vi "DAQ Message Loop.vi"(8 "error in (no error)":errorcluster, 11 "Message Queues":T1) -> (0 "error out":errorcluster)   [LabVIEW 2018]
doc: "Message loop for handling messages pertaining to the acquisition of data from the hardware."
uses:
  <vilib>/Utility/error.llb/Error Cluster From Error Code.vi
  Hardware Configuration.ctl
  DAQ/DAQ Write.lvlib
  support/Message Queue/Message Queue.lvlib
  support/Message Queue/Enqueue Message (Single).vi
  <vilib>/ErrorRing/Error Ring.xnode
  Write State.ctl
  Write Settings Dialog.vi
  Acquisition/Task Cluster.ctl
  support/Message Queue/Message Cluster.ctl
  controls/Queue and Message Cluster.ctl
  DAQ.lvlib
  Main/Main Queue Cluster.ctl
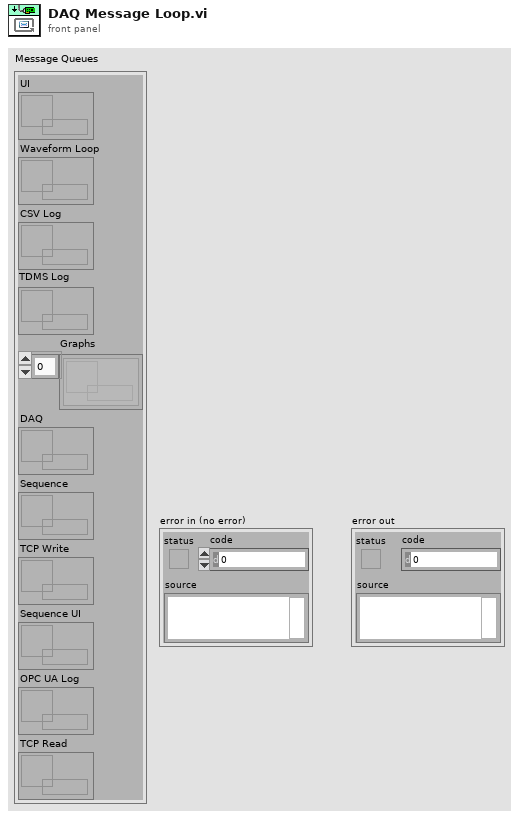
[diagram p1: front panel]
types:
  T1 = typedef "Main Queue Cluster.ctl" = cluster{"UI":refnum<queue>, "Waveform Loop":refnum<queue>, "CSV Log":refnum<queue>, "TDMS Log":refnum<queue>, "Graphs":refnum<queue>[], "DAQ":refnum<queue>, "Sequence":refnum<queue>, "TCP Write":refnum<queue>, "Sequence UI":refnum<queue>, "OPC UA Log":refnum<queue>, "TCP Read":refnum<queue>}
  T2 = typedef "DAQ.lvlib/DAQ Write.lvlib/Hardware Configuration.ctl" = cluster{"Tasks":T3[]}
  T3 = typedef "Task Cluster.ctl" = cluster{"DAQmx Task":refnum<k21>, "Read-Write Radio":enum32{"Read", "Write"}}
  T4 = typedef "Queue and Message Cluster.ctl" = cluster{"return Message Queue":refnum<queue>, "Message":string, "Variant":variant}
  T5 = typedef "Write State.ctl" = enum16{"Idle", "Writting"}
  T6 = typedef "Message Queue.lvlib/Message Cluster.ctl" = cluster{"Message":string, "Message Data":variant}
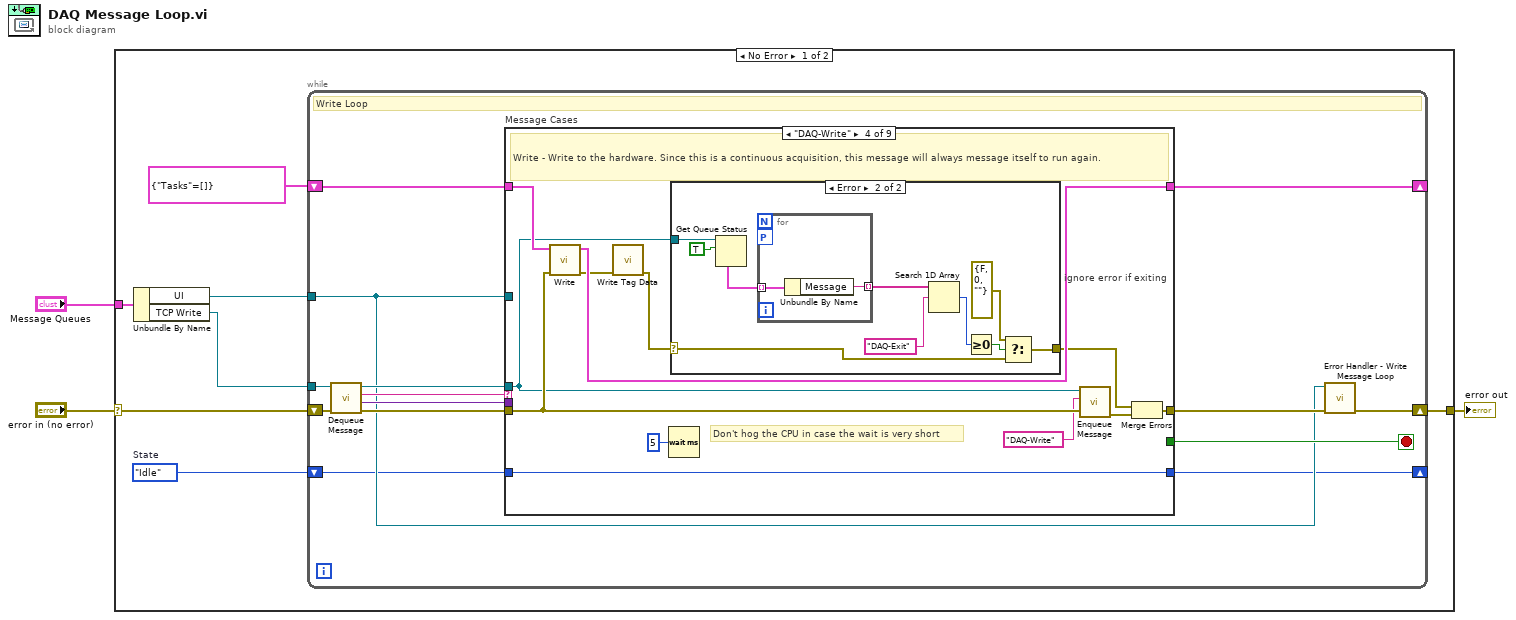
[diagram p0: block diagram]
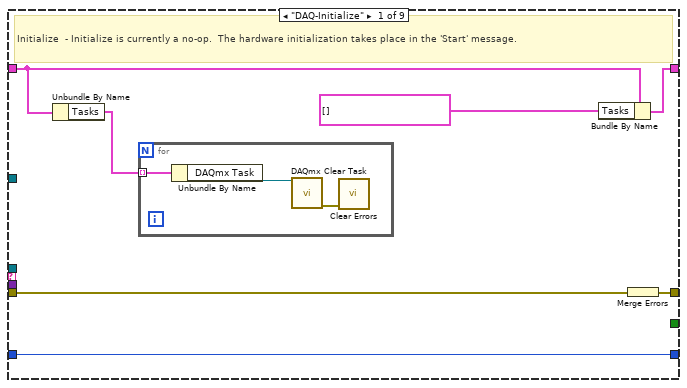
[diagram p2: hidden frame]
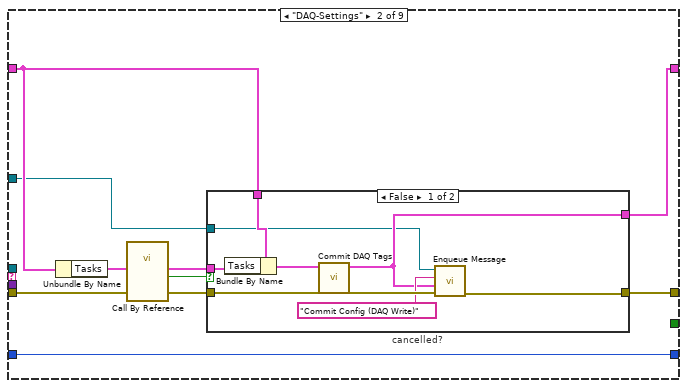
[diagram p3: hidden frame]
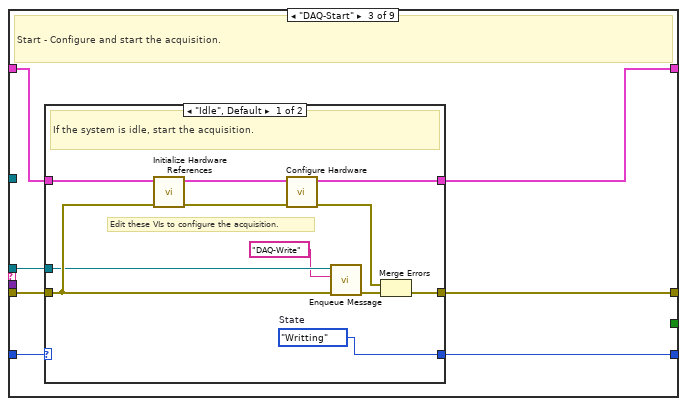
[diagram p5: hidden frame]
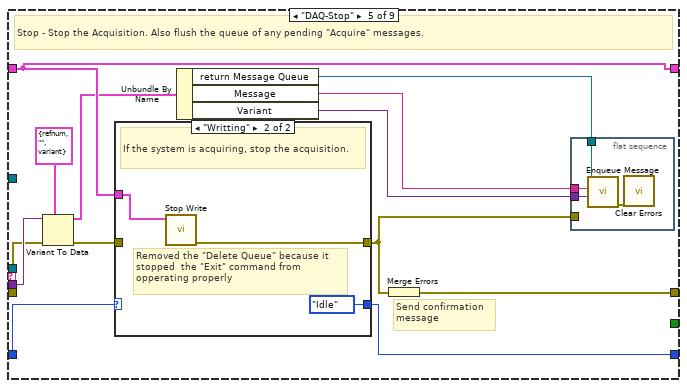
[diagram p8: hidden frame]
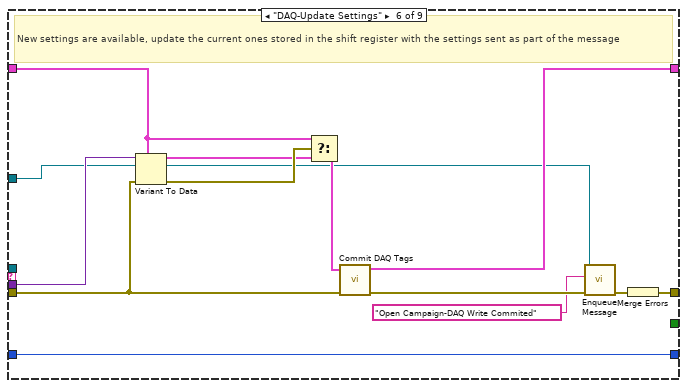
[diagram p10: hidden frame]
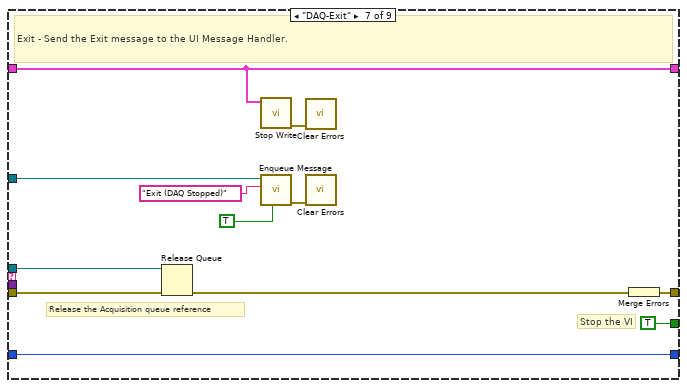
[diagram p11: hidden frame]
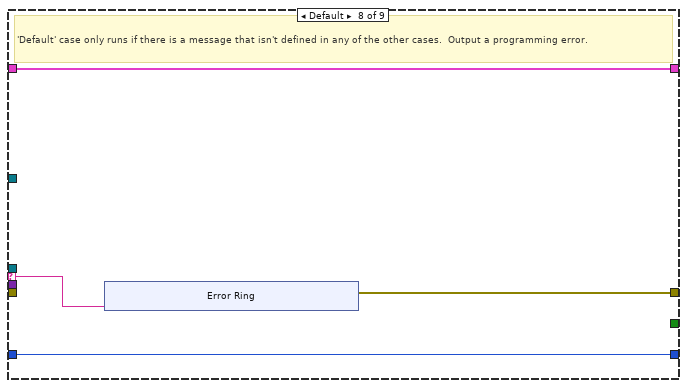
[diagram p12: hidden frame]
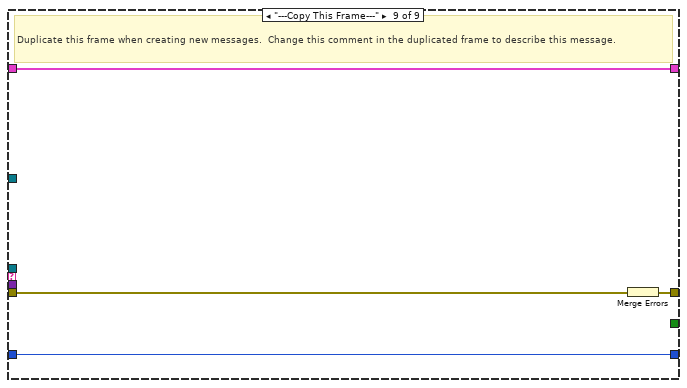
[diagram p13: hidden frame]
diagram:
  n1 = case shown="No Error" "error in (no error)" {
    selector: "error in (no error)" -> [w5 w164]
    tunnel: "Message Queues" -> [w10 _]
    tunnel: [w9 w164] -> w2
    frame No Error {
      w7 = Write_State."Idle"  # State
      n2 = Unbundle By Name(w10) -> ("UI"=w8:refnum<queue>, "TCP Write"=w4:refnum<queue>)
      n3 = while {
        tunnel: w4 -> [w16]
        shift-right: [w23] -> _
        shift-left: T2 {"Tasks"=[]} ("Data Cluster") -> [w24]
        shift-right: [w14] -> w9
        shift-left: w5 -> [w21]
        tunnel: w8 -> [w13]
        shift-right: [w11] -> _
        shift-left: w7 -> [w12]
        stop <- w22 stop-if-true
        # "Write Loop"
        n4 = call "Dequeue Message.vi"("error in (no error)"=w21, "Message Queue"=w16) -> ("error out"=w20:errorcluster, "Message Data"=w18:variant, "Message"=w19:string, "dup Message Queue"=w17:refnum<queue>)  [unwired: 6 in]
        n5 = case "Message Cases" shown="\"DAQ-Write\"" w19 {
          selector: w19 -> [_ _ _ _ _ _ _ w151 _]
          tunnel: w17 -> [_ _ w59 w79 _ _ w141 _ _]
          tunnel: w20 -> [w30 w42 w60 w86 w107 w128 w145 _ w163]
          tunnel: [w31 w36 w62 w88 w114 w136 w147 w150 w161] -> w15
          tunnel: w24 -> [w27 w40 w61 w84 w113 w132 w140 w152 w162]
          tunnel: [w28 w39 w58 w85 w113 w129 w140 w152 w162] -> w23
          tunnel: [_ _ _ _ _ _ TRUE _ _] -> w22
          tunnel: w18 -> [_ _ _ _ w109 w135 _ _ _]
          tunnel: w13 -> [_ w35 _ _ _ w125 w146 _ _]
          tunnel: w12 -> [w29 w44 w57 w82 w112 w131 w139 w149 w160]
          tunnel: [w29 w44 w56 w82 w111 w131 w139 w149 w160] -> w11
          frame "DAQ-Initialize" {
            # "Initialize  - Initialize is currently a no-op.  The hardware initialization takes place in the 'Start' message."
            n6 = Unbundle By Name(w27) -> ("Tasks"=w26:T3[])
            n7 = for {
              tunnel: w26 -> [w34] mode=indexing
              n8 = Unbundle By Name(w34) -> ("DAQmx Task"=w33:refnum<k21>)
              n9 = call <vilib>:"DAQmx Clear Task.vi"("task in"=w33) -> ("error out"=w32:errorcluster)  [unwired: 14 in]
              n10 = call <vilib>:"Clear Errors.vi"("error in (no error)"=w32) -> ()  [unwired: 5 in, 2 out]
            }
            n11 = Bundle By Name(cluster=w27, "Tasks"=T3[] []) -> (w28:T2)
            n12 = Merge Errors(w30) -> (w31:errorcluster)
          }
          frame "DAQ-Settings" {
            n13 = Unbundle By Name(w40) -> ("Tasks"=w41:T3[])
            n14 = call-by-ref "?"("error in (no error)"=w42, "Tasks in"=w41) -> ("error out"=w37:errorcluster, "cancelled"=w38:bool, "Tasks out"=w43:T3[])  [unwired: 9 in, 2 out]
            n15 = case "cancelled?" shown="False" w38 {
              tunnel: w43 -> [w53 _]
              tunnel: w40 -> [w52 w55]
              tunnel: [w47 w55] -> w39
              tunnel: w37 -> [w50 w54]
              tunnel: [w46 w54] -> w36
              tunnel: w35 -> [w45 _]
              frame False {
                n16 = Bundle By Name(cluster=w52, "Tasks"=w53) -> (w51:T2)
                n17 = call "Commit DAQ Tags.vi"("error in (no error)"=w50, "DAQ State in"=w51) -> ("error out"=w49:errorcluster, "DAQ State out"=w47:T2)  [unwired: 8 in]
                n18 = call-poly "Enqueue Message.vi"("error in (no error)"=w49, "Message Data"=w47, "Message"="Commit Config (DAQ Write)", "Message Queue"=w45) -> ("error out"=w46:errorcluster)  [unwired: 6 in, 1 out]
              }
              frame True {
              }
            }
          }
          frame "DAQ-Start" {
            # "Start - Configure and start the acquisition."
            n19 = case shown="\"Idle\", Default" w57 {
              selector: w57 -> [_ w74]
              tunnel: [w73 w76] -> w62
              tunnel: w61 -> [w72 w75]
              tunnel: w60 -> [w71 w76]
              tunnel: w59 -> [w69 _]
              tunnel: [w65 w75] -> w58
              tunnel: [w63 w74] -> w56
              frame "Idle", Default {
                w63 = Write_State."Writting"  # State
                # "Edit these VIs to configure the acquisition."
                # "If the system is idle, start the acquisition."
                n20 = call "Initialize Hardware References.vi"("error in (no error)"=w71, "Hardware Resources in"=w72) -> ("error out"=w68:errorcluster, "Hardware Resources out"=w66:T2)  [unwired: 8 in]
                n21 = call "Configure Hardware.vi"("error in (no error)"=w68, "Hardware Resources in"=w66) -> ("error out"=w67:errorcluster, "Hardware Resources out"=w65:T2)  [unwired: 8 in]
                n22 = call-poly "Enqueue Message.vi"("error in (no error)"=w71, "Message"="DAQ-Write", "Message Queue"=w69) -> ("error out"=w70:errorcluster)  [unwired: 7 in, 1 out]
                n23 = Merge Errors(w67, w70) -> (w73:errorcluster)
              }
              frame "Writting" {
              }
            }
          }
          frame "DAQ-Write" {
            # "Don't hog the CPU in case the wait is very short"
            # "Write - Write to the hardware. Since this is a continuous acquisition, this message will always message itself to run again."
            n24 = call "Write.vi"("error in (no error)"=w86, "Hardware Resources in"=w84) -> ("error out"=w81:errorcluster, "Hardware Resources out"=w85:T2)  [unwired: 8 in]
            n25 = call "Write Tag Data.vi"("error in (no error)"=w81) -> ("error out"=w78:errorcluster)  [unwired: 10 in]
            n26 = Wait (ms)(milliseconds to wait=u32 5) -> ()  [unwired: 1 out]
            n27 = case "ignore error if exiting" shown="Error" w78 {
              selector: w78 -> [w89 w92]
              tunnel: w79 -> [_ w99]
              tunnel: [w89 w91] -> w77
              frame No Error {
              }
              frame Error {
                n28 = Get Queue Status(queue=w99, return elements? (F)=TRUE) -> (elements=w96:T6[])  [unwired: 1 in, 7 out]
                n29 = for {
                  tunnel: w96 -> [w101] mode=indexing
                  tunnel: [w100] -> w95 mode=indexing
                  workers-P: _ -> [_]
                  n30 = Unbundle By Name(w101) -> ("Message"=w100:string)
                }
                n31 = Search 1D Array(1D array=w95, element="DAQ-Exit") -> (index of element=w94:i32)  [unwired: 1 in]
                n32 = Greater Or Equal To 0?(x=w94) -> (x >= 0?=w93:bool)
                n33 = Select(t=errorcluster {"status"=FALSE, "code"=0, "source"=""}, s=w93, f=w92) -> (s? t:f=w91:errorcluster)
              }
            }
            n34 = call-poly "Enqueue Message.vi"("error in (no error)"=w86, "Message"="DAQ-Write", "Message Queue"=w79) -> ("error out"=w87:errorcluster)  [unwired: 7 in, 1 out]
            n35 = Merge Errors(w77, w87) -> (w88:errorcluster)
          }
          frame "DAQ-Stop" {
            # "Send confirmation\nmessage"
            # "Stop - Stop the Acquisition. Also flush the queue of any pending \"Acquire\" messages."
            n36 = Variant To Data(error in=w107, type=T4 {"return Message Queue"=refnum, "Message"="", "Variant"=variant} ("Queue and Message"), Variant=w109) -> (data=w106:T4, error out=w108:errorcluster)
            n37 = case shown="\"Writting\"" w112 {
              selector: w112 -> [w120 _]
              tunnel: w108 -> [w119 _]
              tunnel: w113 -> [_ w123]
              tunnel: [w120 Write_State."Idle" ("State")] -> w111
              tunnel: [w119 w121] -> w102
              frame "Idle", Default {
                # "The system is already idle. Ignore the \"Stop\" message."
              }
              frame "Writting" {
                # "Removed the \"Delete Queue\" because it\nstopped  the \"Exit\" command from \nopperating properly"
                # "If the system is acquiring, stop the acquisition."
                n38 = call "Stop Write.vi"("Hardware Resources in"=w123) -> ("error out"=w121:errorcluster)  [unwired: 10 in]
              }
            }
            n39 = Unbundle By Name(w106) -> ("return Message Queue"=w105:refnum<queue>, "Message"=w104:string, "Variant"=w103:variant)
            n40 = Merge Errors(w102) -> (w114:errorcluster)
            n41 = flat-sequence {
              tunnel: w105 -> [w118]
              tunnel: w104 -> [w117]
              tunnel: w103 -> [w116]
              tunnel: w102 -> [_]
              frame #0 {
                n42 = call-poly "Enqueue Message.vi"("Message Data"=w116, "Message"=w117, "Message Queue"=w118) -> ("error out"=w115:errorcluster)  [unwired: 7 in, 1 out]
                n43 = call <vilib>:"Clear Errors.vi"("error in (no error)"=w115) -> ()  [unwired: 5 in, 2 out]
              }
            }
          }
          frame "DAQ-Update Settings" {
            # "New settings are available, update the current ones stored in the shift register with the settings sent as part of the message"
            n44 = Variant To Data(error in=w128, type=w132, Variant=w135) -> (data=w133:T2, error out=w134:errorcluster)
            n45 = Select(t=w132, s=w134, f=w133) -> (s? t:f=w130:T2)
            n46 = call "Commit DAQ Tags.vi"("error in (no error)"=w128, "DAQ State in"=w130) -> ("error out"=w127:errorcluster, "DAQ State out"=w129:T2)  [unwired: 8 in]
            n47 = call-poly "Enqueue Message.vi"("error in (no error)"=w127, "Message"="Open Campaign-DAQ Write Commited", "Message Queue"=w125) -> ("error out"=w126:errorcluster)  [unwired: 7 in, 1 out]
            n48 = Merge Errors(w126) -> (w136:errorcluster)
          }
          frame "DAQ-Exit" {
            # "Release the Acquisition queue reference"
            # "Stop the VI"
            # "Exit - Send the Exit message to the UI Message Handler."
            n49 = Release Queue(queue=w141, error in (no error)=w145) -> (error out=w142:errorcluster)  [unwired: 1 in, 2 out]
            n50 = call "Stop Write.vi"("Hardware Resources in"=w140) -> ("error out"=w138:errorcluster)  [unwired: 10 in]
            n51 = call-poly "Enqueue Message.vi"("Priority Message? (F)"=TRUE, "Message"="Exit (DAQ Stopped)", "Message Queue"=w146) -> ("error out"=w137:errorcluster)  [unwired: 7 in, 1 out]
            n52 = call <vilib>:"Clear Errors.vi"("error in (no error)"=w138) -> ()  [unwired: 5 in, 2 out]
            n53 = call <vilib>:"Clear Errors.vi"("error in (no error)"=w137) -> ()  [unwired: 5 in, 2 out]
            n54 = Merge Errors(w142) -> (w147:errorcluster)
          }
          frame Default {
            # "'Default' case only runs if there is a message that isn't defined in any of the other cases.  Output a programming error."
            n55 = xnode "Error Ring"("parameter 0"=w151) -> ("error out"=w150:errorcluster)
          }
          frame "---Copy This Frame---" {
            # "Duplicate this frame when creating new messages.  Change this comment in the duplicated frame to describe this message."
            n56 = Merge Errors(w163) -> (w161:errorcluster)
          }
        }
        n57 = call "Error Handler - Write Message Loop.vi"("error in (no error)"=w15, "Message Queue"=w13) -> ("dup error in"=w14:errorcluster)  [unwired: 8 in, 1 out]
      }
    }
    frame Error {
    }
  }
  "error out" <- w2
